vi "Init Server.vi"(5 "EventLogger":refnum<class "EventLoggingService.lvclass">, 7 "SequenceCountService":refnum<class "SequenceCountService.lvclass">, 8 "error in (no error)":errorcluster, 9 "Bind Port":u16, 10 "Bind Address":string, 11 "Node ID":u32) -> (0 "error out":errorcluster, 3 "TCPMessaging out":refnum<class "TCPMessaging.lvclass">)   [LabVIEW 2020, in "Vecto.lvlib" / "TCPMessaging.lvclass"]
uses:
  TCPMessaging.lvclass
  SequenceCountService/SequenceCountService.lvclass
  EventLoggingService/EventLoggingService.lvclass
  TCP Mode.ctl
  Event Level.ctl
  TCPMessaging.lvclass/TCPMessaging.ctl
  EventLoggingService/EventLoggingService.lvclass/EventLoggingService.ctl
  <vilib>/Utility/error.llb/Error Cluster From Error Code.vi
  EventLogHandler/EventLogHandler.lvclass
  Vecto.lvlib
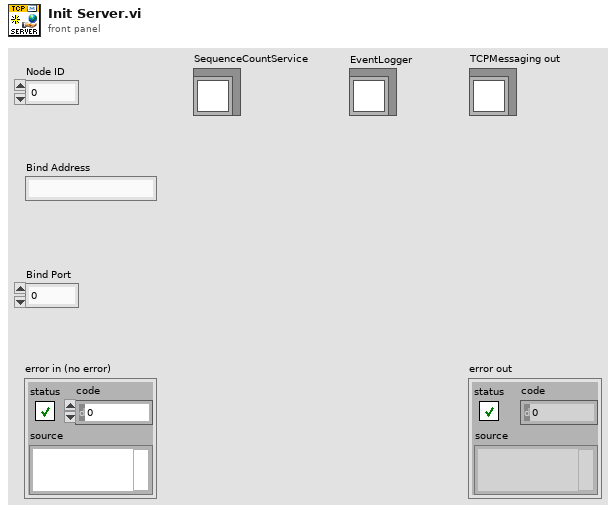
[diagram p1: front panel]
types:
  T1 = typedef "Vecto.lvlib/Event Level.ctl" = enum16{"Debug", "Info", "Warning", "Error"}
  T2 = typedef "Vecto.lvlib/TCPMessaging.lvclass/TCP Mode.ctl" = enum16{"Client", "Server"}
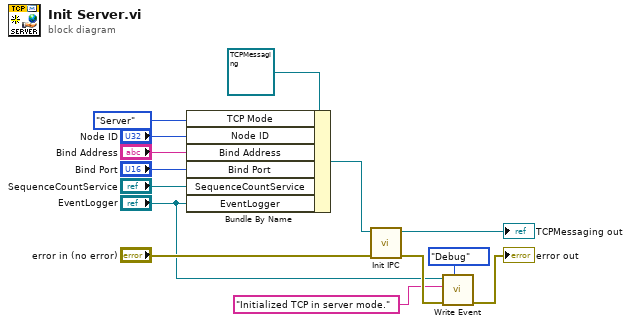
[diagram p0: block diagram]
diagram:
  n1 = Bundle By Name(cluster=refnum<class "TCPMessaging.lvclass"> refnum ("TCPMessaging in"), "TCP Mode"=TCP_Mode."Server", "Node ID"="Node ID", "Bind Address"="Bind Address", "Bind Port"="Bind Port", "SequenceCountService"="SequenceCountService", "EventLogger"="EventLogger") -> (w8:refnum<class "TCPMessaging.lvclass">)
  n2 = call "Init IPC.vi"("error in (no error)"="error in (no error)", "TCPMessaging in"=w8) -> ("error out"=w9:errorcluster, "TCPMessaging out"=→"TCPMessaging out":refnum<class "TCPMessaging.lvclass">)  [unwired: 8 in]
  n3 = call "Write Event.vi"("Event Level (Info)"=Event_Level."Debug", "error in (no error)"=w9, "Message"="Initialized TCP in server mode.", "EventLoggingService in"="EventLogger") -> ("error out"=→"error out":errorcluster)  [unwired: 6 in, 1 out]
